vi "GCMPlugin_Stop.vi"(8 "error in (no error)":errorcluster, 11 "_LVCMPlugin in":refnum<class "GCMPlugin.lvclass">) -> (0 "error out":errorcluster, 3 "_LVCMPlugin out":refnum<class "GCMPlugin.lvclass">)   [LabVIEW 2014, in "GCMPlugin.lvclass"]
uses:
  GCMPlugin/GCMPlugin.lvclass
  GCMPlugin/GCMPlugin.lvclass/GCMPlugin.ctl
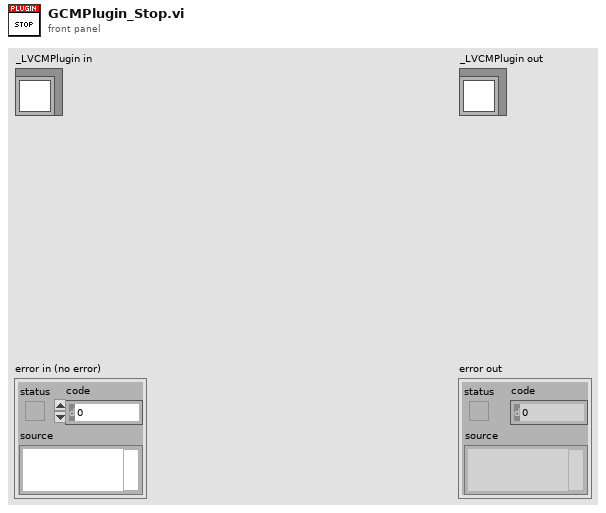
[diagram p1: front panel]
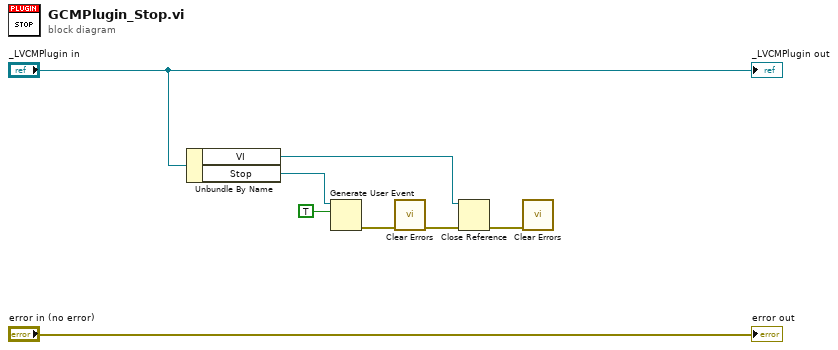
[diagram p0: block diagram]
diagram:
  n1 = Unbundle By Name("_LVCMPlugin in") -> ("VI"=w5:refnum<vi>, "Stop"=w7:refnum<user-event>)
  n2 = Generate User Event(user event=w7, event data cluster=TRUE ("event data")) -> (error out=w2:errorcluster)  [unwired: 2 in, 1 out]
  n3 = call <vilib>:"Clear Errors.vi"("error in (no error)"=w2) -> ("error out"=w1:errorcluster)  [unwired: 5 in, 1 out]
  n4 = Close Reference(reference=w5, error in (no error)=w1) -> (error out=w4:errorcluster)
  n5 = call <vilib>:"Clear Errors.vi"("error in (no error)"=w4) -> ()  [unwired: 5 in, 2 out]
  "error out" <- "error in (no error)"
  "_LVCMPlugin out" <- "_LVCMPlugin in"
